vi "Get_Calbration_times.vi"() -> (0 "Seconds since 1904":dbl[](array[numeric]) format="%.2f", 1 "Calib Filenames":path[](array[path]))   [LabVIEW 2012]
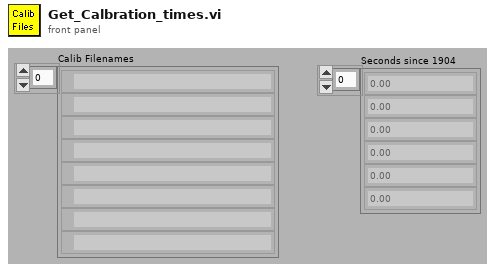
[diagram p1: front panel]
types:
  T1 = enum32{"existing file", "new file", "new or existing file", "existing dir", "new dir", "new or existing dir", "existing file (use LLBs)", "new file (use LLBs)", "new or existing file (use LLBs)", "new or existing file or directory (use LLBs)"}
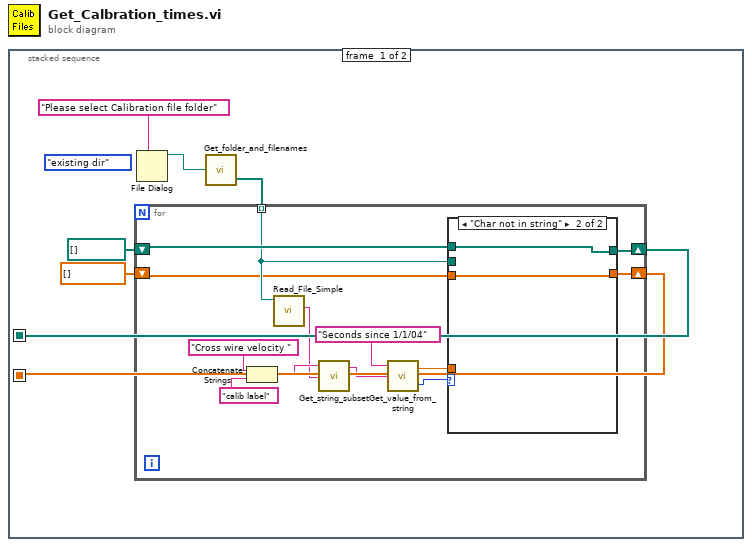
[diagram p0: block diagram]
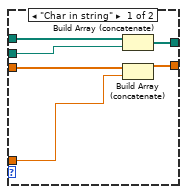
[diagram p2: hidden frame]
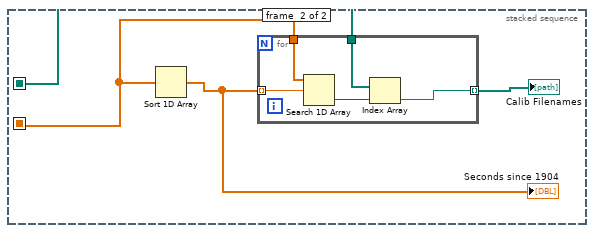
[diagram p3: hidden frame]
diagram:
  n1 = stacked-sequence {
    seq-local: [w2 _] -> [_ w30]
    seq-local: [w1 _] -> [_ w31]
    frame #0 {
      (unwired) T1."existing dir" ("select mode (2)")
      n2 = File Dialog(7:"Please select Calibration file folder" ("prompt")) -> (3:w6:path)  [unwired: 6 in, 3 out]
      n3 = call "Get_folder_and_filenames.vi"("file path (dialog if empty)"=w6) -> ("Files"=w5:path[])  [unwired: 1 out]
      n4 = for {
        shift-right: [w11] -> w2
        shift-left: path[] [] -> [w13]
        shift-right: [w10] -> w1
        shift-left: dbl[] [] -> [w9]
        tunnel: w5 -> [w12] mode=indexing
        n5 = Concatenate Strings("Cross wire velocity ", "calib label") -> (w18:string)
        n6 = call "Read_File_Simple.vi"("Filename"=w12) -> ("string"=w17:string)  [unwired: 4 in, 5 out]
        n7 = call "Get_string_subset.vi"("String to split"=w17, "File Label"=w18) -> ("Output string"=w15:string)  [unwired: 2 in, 1 out]
        n8 = call "Get_value_from_string.vi"("Input string"=w15, "Variable name"="Seconds since 1/1/04") -> ("Status"=w14:enum16{"Char in string", "Char not in string"}, "Value"=w8:dbl)  [unwired: 1 in]
        n9 = case shown="\"Char not in string\"" w14 {
          tunnel: w13 -> [w26 w28]
          tunnel: w12 -> [w25 _]
          tunnel: [w24 w28] -> w11
          tunnel: [w23 w27] -> w10
          tunnel: w9 -> [w22 w27]
          tunnel: w8 -> [w21 _]
          frame "Char in string" {
            n10 = Build Array (concatenate)(w26, w25) -> (w24:path[])
            n11 = Build Array (concatenate)(w22, w21) -> (w23:dbl[])
          }
          frame "Char not in string" {
          }
        }
      }
    }
    frame #1 {
      n12 = Sort 1D Array(array=w31) -> (sorted array=w32:dbl[])
      "Seconds since 1904" <- w32
      n13 = for {
        tunnel: w31 -> [w37]
        tunnel: w32 -> [w36] mode=indexing
        tunnel: w30 -> [w35]
        tunnel: [w34] -> w29 mode=indexing
        n14 = Search 1D Array(1D array=w37, element=w36) -> (index of element=w33:i32)  [unwired: 1 in]
        n15 = Index Array(array=w35, index=w33) -> (element=w34:path)
      }
      "Calib Filenames" <- w29
    }
  }
